vi "Register_Web_Services.vi"(8 "error in":errorcluster, 10 "eng_installPath":string, 11 "source path":path) -> (0 "error out":errorcluster, 2 "Pre_Uninstall_Step":refnum<class "IB_Post_Install_Step.lvclass">, 3 "Post_Install_Step":refnum<class "IB_Post_Install_Step.lvclass">)   [LabVIEW 2020, in "IB_Source.lvclass"]
uses:
  <vilib>/AppBuilder/IB_Classes/Source/IB_Source.lvclass
  <vilib>/AppBuilder/IB_Classes/Source/IB_Source.lvclass/IB_Source.ctl
  <vilib>/AppBuilder/IB_Classes/Post_Install_Step/IB_Post_Install_Step.lvclass
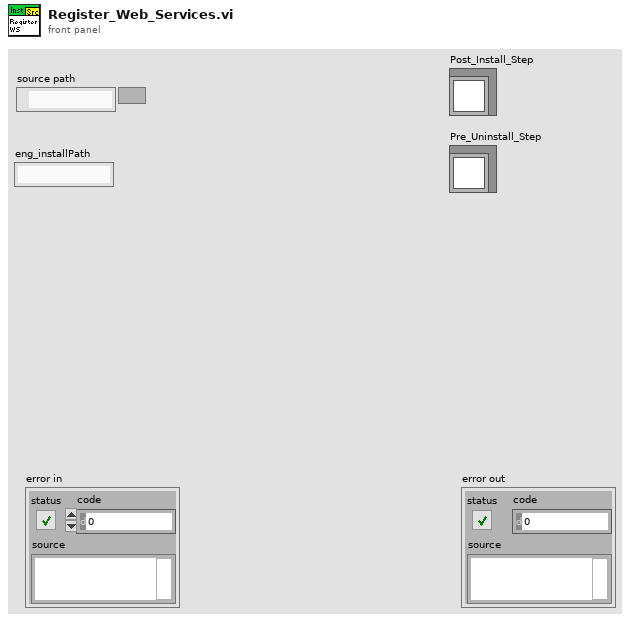
[diagram p1: front panel]
types:
  T1 = typedef "IB_Post_Install_Step.ctl" = cluster{"command":path, "arg":string}
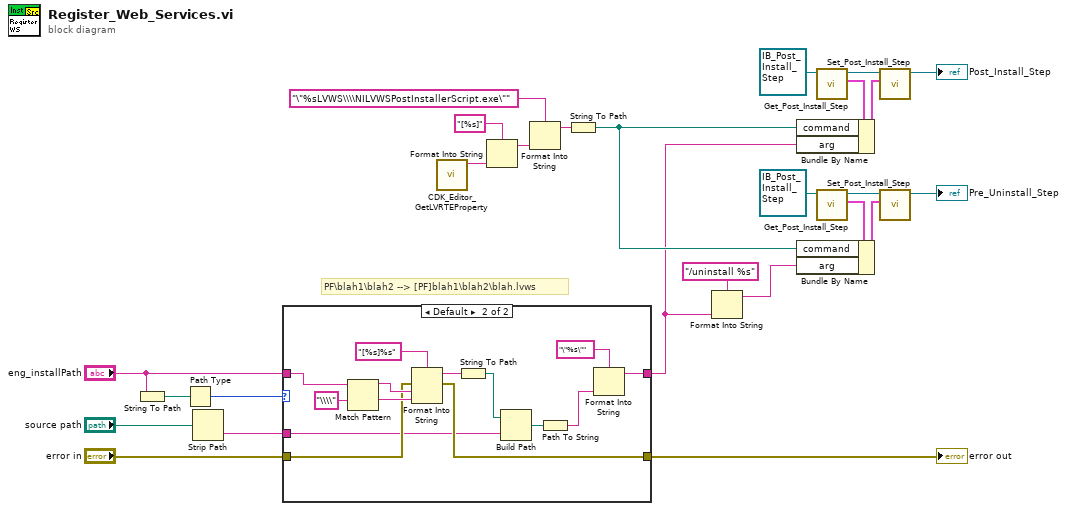
[diagram p0: block diagram]
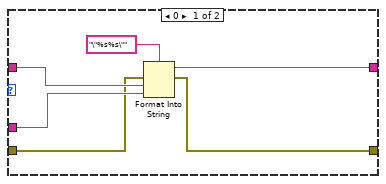
[diagram p2: hidden frame]
diagram:
  # "PF\\blah1\\blah2 --> [PF]blah1\\blah2\\blah.lvws"
  n1 = String To Path(string="eng_installPath") -> (path=w17:path)
  n2 = Path Type(1:w17) -> (0:w16:i16)
  n3 = Strip Path(path="source path") -> (name=w15:string)  [unwired: 1 out]
  n4 = case shown="Default" w16 {
    tunnel: "eng_installPath" -> [w30 w42]
    tunnel: [w29 w39] -> w8
    tunnel: w15 -> [w31 w36]
    tunnel: "error in" -> [w27 w41]
    tunnel: [w28 w40] -> w4
    frame 0 {
      n5 = Format Into String(format string="\"%s%s\"", error in=w27, w30, w31) -> (resulting string=w29:string, error out=w28:errorcluster)  [unwired: 1 in]
    }
    frame Default {
      n6 = Match Pattern(string=w42, regular expression="\\\\") -> (before substring=w45:string, after substring=w46:string)  [unwired: 3 out]
      n7 = Format Into String(format string="[%s]%s", error in=w41, w45, w46) -> (resulting string=w35:string, error out=w40:errorcluster)  [unwired: 1 in]
      n8 = String To Path(string=w35) -> (path=w37:path)
      n9 = Build Path(base path=w37, name or relative path=w36) -> (appended path=w34:path)
      n10 = Path To String(path=w34) -> (string=w33:string)
      n11 = Format Into String(format string="\"%s\"", w33) -> (resulting string=w39:string)  [unwired: 2 in, 1 out]
    }
  }
  "error out" <- w4
  n12 = call <resource>:"CDK_Editor_GetLVRTEProperty.vi"() -> ("LVRTE property"=w23:string)  [unwired: 11 out]
  n13 = Format Into String(format string="[%s]", w23) -> (resulting string=w25:string)  [unwired: 2 in, 1 out]
  n14 = Format Into String(format string="\"%sLVWS\\\\NILVWSPostInstallerScript.exe\"", w25) -> (resulting string=w26:string)  [unwired: 2 in, 1 out]
  n15 = String To Path(string=w26) -> (path=w10:path)
  n16 = Format Into String(format string="/uninstall %s", w8) -> (resulting string=w7:string)  [unwired: 2 in, 1 out]
  n17 = call <vilib>:"Get_Post_Install_Step.vi"("IB_Post_Install_Step in"=refnum<class "IB_Post_Install_Step.lvclass"> refnum ("Post_Install_Steps")) -> ("data"=w19:T1, "IB_Post_Install_Step out"=w20:refnum<class "IB_Post_Install_Step.lvclass">)  [unwired: 1 in, 8 out]
  n18 = Bundle By Name(cluster=w19, "command"=w10, "arg"=w8) -> (w18:T1)
  n19 = call <vilib>:"Get_Post_Install_Step.vi"("IB_Post_Install_Step in"=refnum<class "IB_Post_Install_Step.lvclass"> refnum ("Post_Install_Steps")) -> ("data"=w13:T1, "IB_Post_Install_Step out"=w12:refnum<class "IB_Post_Install_Step.lvclass">)  [unwired: 1 in, 8 out]
  n20 = Bundle By Name(cluster=w13, "command"=w10, "arg"=w7) -> (w14:T1)
  n21 = call <vilib>:"Set_Post_Install_Step.vi"("data"=w18, "IB_Post_Install_Step in"=w20) -> ("IB_Post_Install_Step out"=→"Post_Install_Step":refnum<class "IB_Post_Install_Step.lvclass">)  [unwired: 1 in, 8 out]
  n22 = call <vilib>:"Set_Post_Install_Step.vi"("data"=w14, "IB_Post_Install_Step in"=w12) -> ("IB_Post_Install_Step out"=→"Pre_Uninstall_Step":refnum<class "IB_Post_Install_Step.lvclass">)  [unwired: 1 in, 8 out]
